vi "Comprar.vi"(8 "error in (no error)":errorcluster, 10 "Pagar":bool, 11 "Soda Actor in":refnum<class "Soda Actor.lvclass">) -> (0 "error out":errorcluster, 3 "Soda Actor out":refnum<class "Soda Actor.lvclass">)   [LabVIEW 2019, in "Soda Actor.lvlib" / "Soda Actor.lvclass"]
uses:
  Soda Actor.lvclass
  C:/Program Files (x86)/National Instruments/LabVIEW 2019/vi.lib/ActorFramework/Actor/Actor.lvclass
  <vilib>/ActorFramework/Actor/Actor.lvclass/Actor.ctl
  Soda Actor.lvclass/Soda Actor.ctl
  UI Actor Messages/Comprar Msg/Comprar Msg.lvclass/Comprar Msg.ctl
  <vilib>/ActorFramework/Message Enqueuer/Message Enqueuer.lvclass/Message Enqueuer.ctl
  <vilib>/ActorFramework/Message Enqueuer/Enqueue.vi
  UI Actor Messages/Comprar Msg/Comprar Msg.lvclass
  C:/Program Files (x86)/National Instruments/LabVIEW 2019/vi.lib/ActorFramework/Message/Message.lvclass
  <vilib>/ActorFramework/Message Priority Queue/Priority Enqueue.vi
  <vilib>/ActorFramework/Actor/Actor.lvclass
panel:
  in  "Cluster":T1
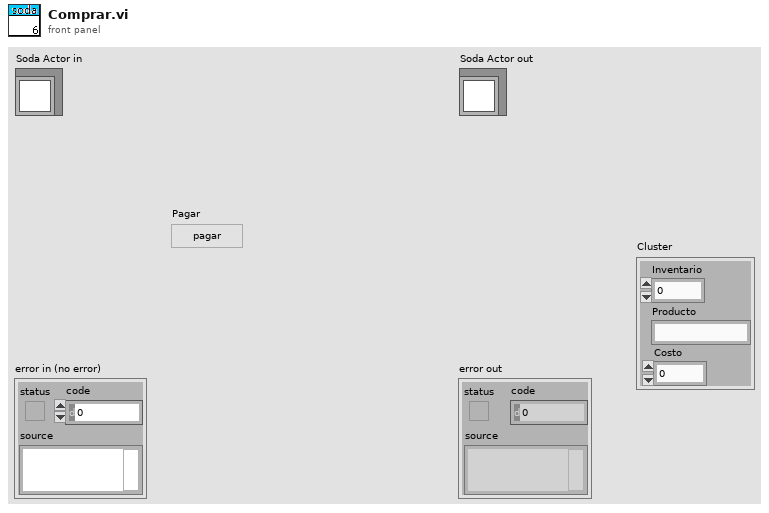
[diagram p1: front panel]
types:
  T1 = cluster{"Inventario":i32, "Producto":string, "Costo":dbl}
  T2 = cluster{"Listaselect[0]":string, "Listaselect[1]":string, "Listaselect[2]":string, "Listaselect[3]":string, "Listaselect[4]":string, "Listaselect[5]":string, "Listaselect[6]":string, "Listaselect[7]":string, "Listaselect[8]":string}
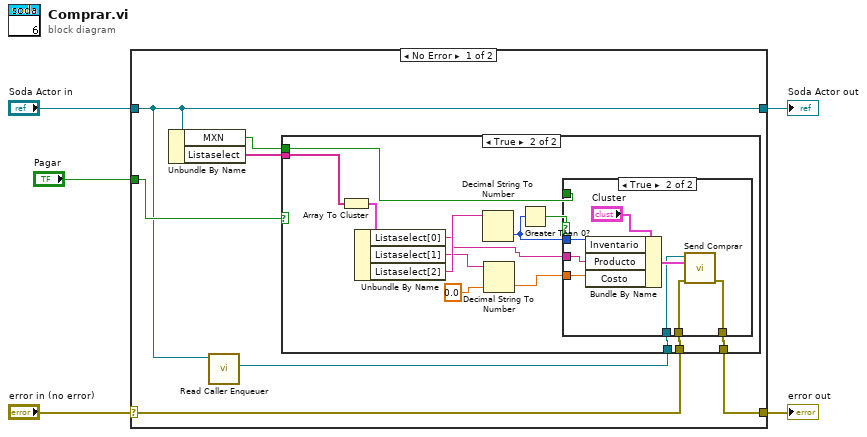
[diagram p0: block diagram]
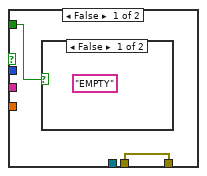
[diagram p3: hidden frame]
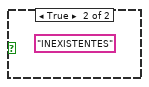
[diagram p4: hidden frame]
diagram:
  n1 = case shown="No Error" "error in (no error)" {
    selector: "error in (no error)" -> [w7 w38]
    tunnel: [w6 w38] -> w4
    tunnel: [w9 w37] -> w2
    tunnel: "Soda Actor in" -> [w9 w37]
    tunnel: "Pagar" -> [w12 _]
    frame No Error {
      n2 = Unbundle By Name(w9) -> ("MXN"=w10:bool, "Listaselect"=w11:string[])
      n3 = call <vilib>:"Read Caller Enqueuer.vi"("Actor"=w9) -> ("Caller Enqueuer"=w8:refnum<class "Message Enqueuer.lvclass">)  [unwired: 10 in]
      n4 = case shown="True" w12 {
        tunnel: w11 -> [_ w26]
        tunnel: w10 -> [_ w23]
        tunnel: w8 -> [_ w16]
        tunnel: w7 -> [w13 w15]
        tunnel: [w13 w14] -> w6
        frame False {
        }
        frame True {
          n5 = Array To Cluster(array=w26) -> (cluster=w25:T2)
          n6 = Unbundle By Name(w25) -> ("Listaselect[0]"=w17:string, "Listaselect[1]"=w20:string, "Listaselect[2]"=w24:string)
          n7 = Decimal String To Number(string=w24) -> (number=w21:i32)  [unwired: 2 in, 1 out]
          n8 = Decimal String To Number(string=w20, default (0L)=0.0) -> (number=w18:dbl)  [unwired: 1 in, 1 out]
          n9 = Greater Than 0?(x=w21) -> (x > 0?=w22:bool)
          n10 = case shown="True" w22 {
            tunnel: w23 -> [w28 _]
            tunnel: w21 -> [_ w36]
            tunnel: w18 -> [_ w33]
            tunnel: w17 -> [_ w34]
            tunnel: w16 -> [_ w31]
            tunnel: w15 -> [w27 w30]
            tunnel: [w27 w29] -> w14
            frame False {
              n11 = case shown="False" w28 {
                frame False {
                  (unwired) "EMPTY"
                }
                frame True {
                  (unwired) "INEXISTENTES"
                }
              }
            }
            frame True {
              n12 = Bundle By Name(cluster="Cluster", "Inventario"=w36, "Producto"=w34, "Costo"=w33) -> (w32:T1)
              n13 = call "Send Comprar.vi"("error in (no error)"=w30, "Cluster"=w32, "Message Enqueuer"=w31) -> ("error out"=w29:errorcluster)  [unwired: 7 in, 1 out]
            }
          }
        }
      }
    }
    frame Error {
    }
  }
  "error out" <- w4
  "Soda Actor out" <- w2
